vi "solar_qtimer Refnum SEQ to QTimer.vi"(1 "QTimers SEQ":refnum<queue>) -> (0 "QTimer Refnum":T1)   [LabVIEW 2018]
doc: "This type casts to the QTimer reference."
uses:
  solar_qtimer_ctl Refnum.ctl
  solar_qtimer_ctl QTimer.ctl
  solar_qtimer_ctl SEQ.ctl
  solar_qtimer_ctl QTimer Settings.ctl
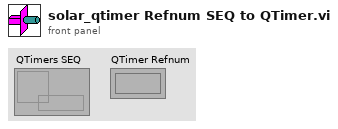
[diagram p1: front panel]
types:
  T1 = typedef "solar_qtimer_ctl Refnum.ctl" = refnum<k1>
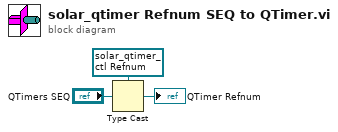
[diagram p0: block diagram]
diagram:
  w1 = T1 refnum items=["qtimer"] ("QTimer Refnum")
  n1 = Type Cast(type=w1, x="QTimers SEQ") -> (*(type *) &x=→"QTimer Refnum":T1)
